vi "VISA_Read_4CHparalelos.vi"() -> ()   [LabVIEW 2019]
uses:
  <vilib>/Instr/_visa.llb/VISA Configure Serial Port (Instr).vi
panel:
  out "Plot 3":dbl[](graph)
  out "Plot 2":dbl[](graph)
  out "Plot 1":dbl[](graph)
  out "Plot 0":dbl[](graph)
  out "Status Read":errorcluster
  out "Buffer Array":dbl[](array[numeric])
  out "Read Buffer":string
  out "Status Serial":errorcluster
  in  "Stop Read":bool
  in  "Start Read":bool
  in  "baud rate (9600)":u32=115200
  in  "data bits (8)":u8=8 min=5 max=8 step=1
  in  "VISA resource name":refnum<visa-resource-name>
  # "Log de Erros"
  # "Conversão Para Inteiro"
  # "Resultado da Leitura"
  # "Controle da porta Serial USB"
  # "Controle da Leitura"
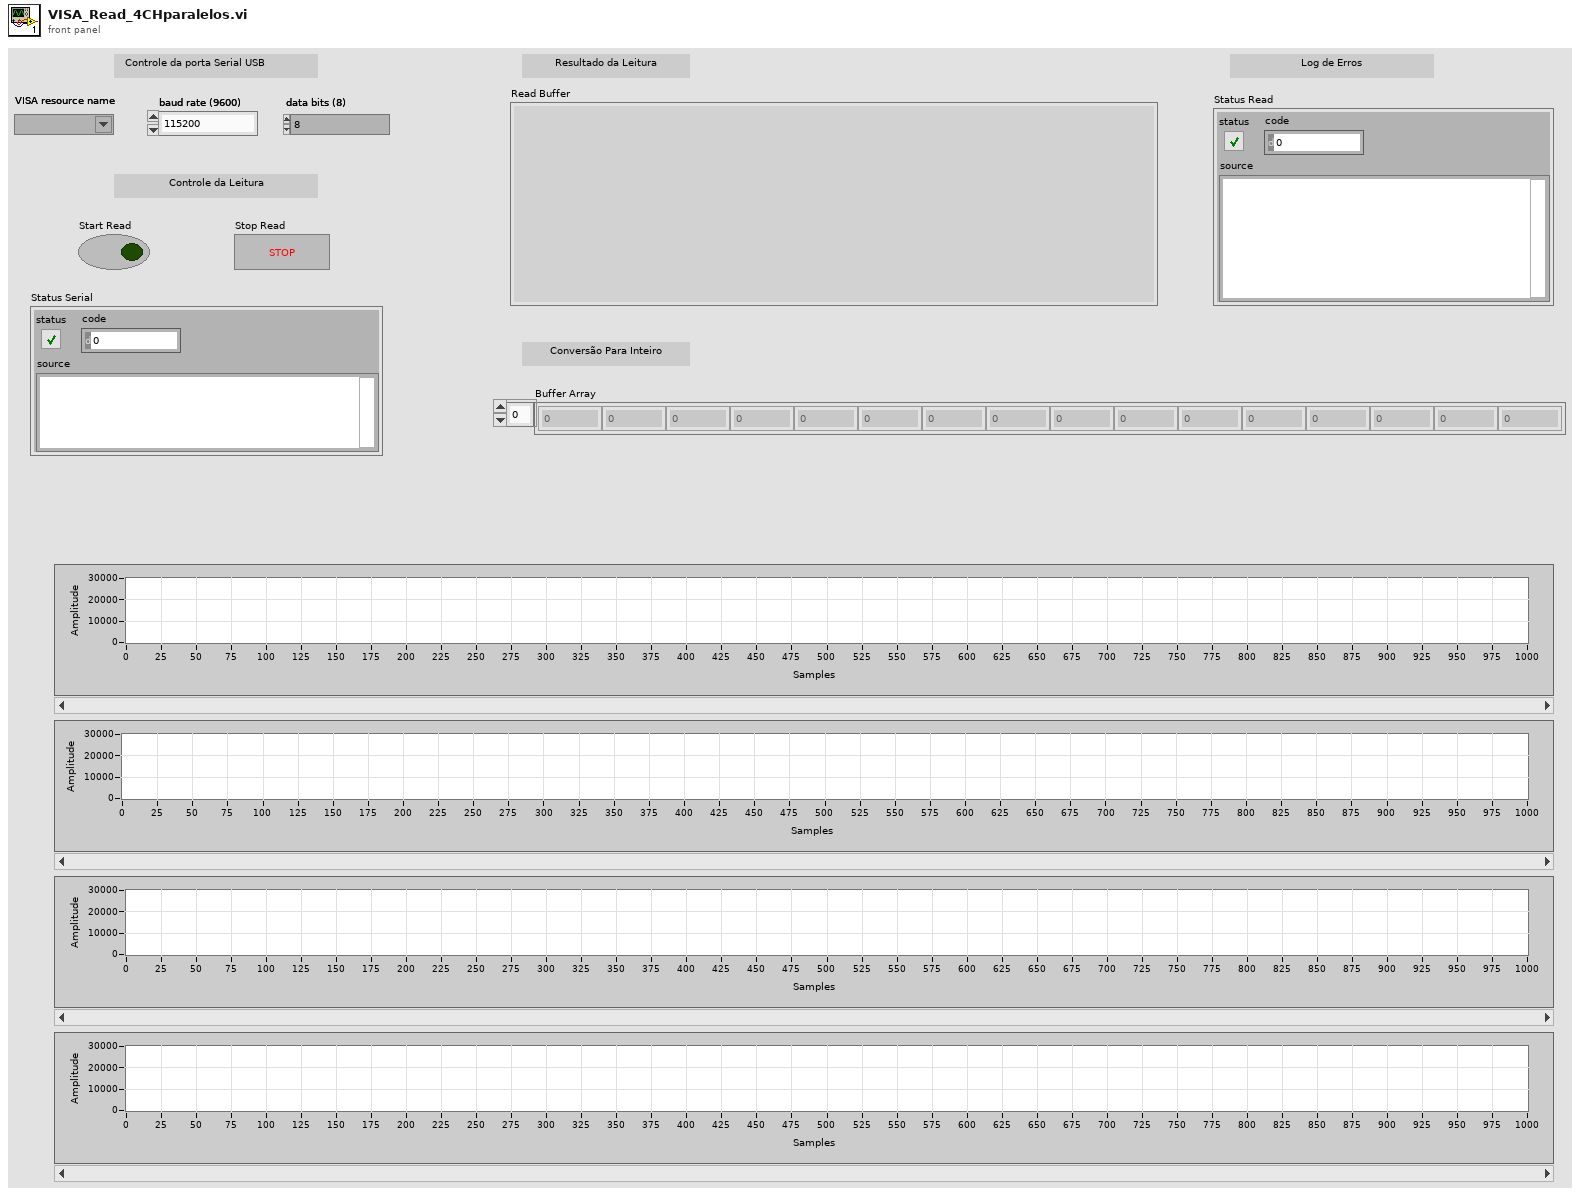
[diagram p1: front panel]
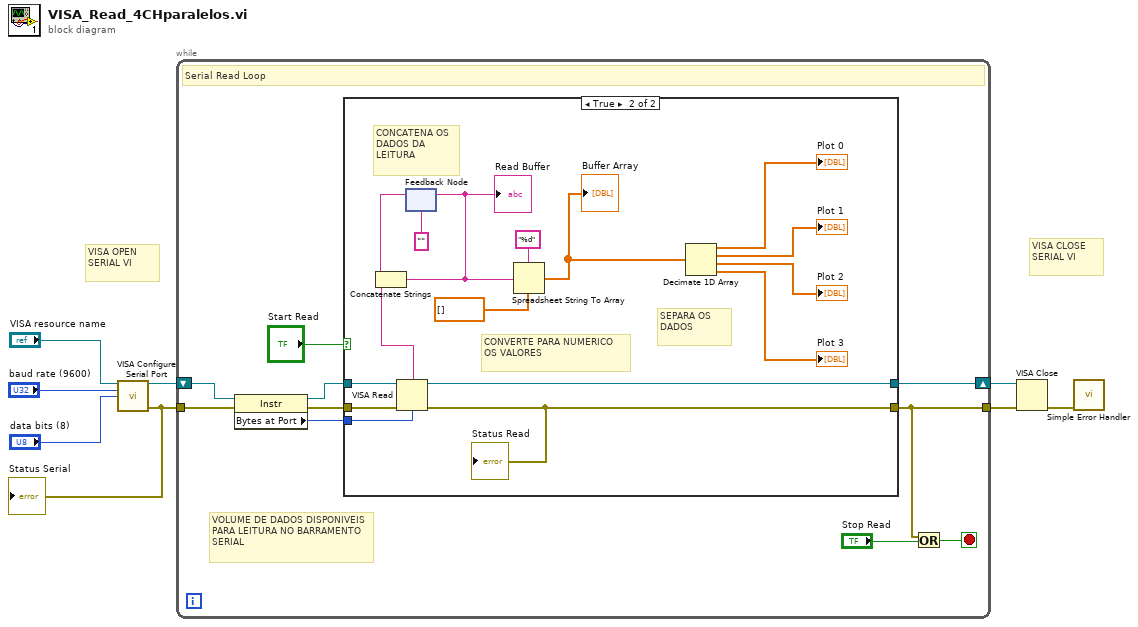
[diagram p0: block diagram]
diagram:
  # "VISA OPEN SERIAL VI"
  # "VISA CLOSE SERIAL VI"
  n1 = call-poly "VISA Configure Serial Port"("VISA resource name"="VISA resource name", "baud rate (9600)"="baud rate (9600)", "data bits (8)"="data bits (8)") -> ("VISA resource name out"=w6:refnum<visa-resource-name>, "error out"=w1:errorcluster)  [unwired: 11 in]
  "Status Serial" <- w1
  n2 = while {
    tunnel: w1 -> [w12]
    tunnel: [w16] -> w7
    shift-right: [w15] -> w5
    shift-left: w6 -> [w13]
    stop <- w14 stop-if-true
    # "VOLUME DE DADOS DISPONIVEIS PARA LEITURA NO BARRAMENTO SERIAL"
    # "Serial Read Loop"
    n3 = property class="Instr"(reference=w13, error in=w12) -> (reference out=w9:refnum<visa-resource-name>, error out=w10:errorcluster, "Bytes at Port"=w11:u32)
    n4 = case shown="True" "Start Read" {
      tunnel: [w19 w36] -> w16
      tunnel: [w20 w33] -> w15
      tunnel: w11 -> [_ w29]
      tunnel: w9 -> [w20 w28]
      tunnel: w10 -> [w19 w27]
      frame False {
        # "OS DADOS SÃO ACUMULADOS NO BUFFER ESPERANDO A PERMISSÃO PARA SER LIDOS"
      }
      frame True {
        # "SEPARA OS DADOS"
        # "CONVERTE PARA NUMERICO OS VALORES"
        # "CONCATENA OS DADOS DA LEITURA"
        n5 = VISA Read(VISA resource name=w28, byte count=w29, error in (no error)=w27) -> (VISA resource name out=w33:refnum<visa-resource-name>, read buffer=w35:string, error out=w36:errorcluster)  [unwired: 1 out]
        "Status Read" <- w36
        n6 = feedback #1("") -> (w30:string)
        n7 = Concatenate Strings(w30, w35) -> (w32:string)
        "Read Buffer" <- w32
        n8 = feedback-in #1(w32) -> ()
        n9 = Spreadsheet String To Array(format string="%d", spreadsheet string=w32, array type (2D Dbl)=dbl[] []) -> (array=w24:dbl[])  [unwired: 1 in]
        "Buffer Array" <- w24
        n10 = Decimate 1D Array(w24) -> (→"Plot 0":dbl[], →"Plot 1":dbl[], →"Plot 2":dbl[], →"Plot 3":dbl[])
      }
    }
    n11 = Or(x=w16, y="Stop Read") -> (x .or. y?=w14:bool)
  }
  n12 = VISA Close(VISA resource name=w5, error in (no error)=w7) -> (error out=w4:errorcluster)
  n13 = call <vilib>:"Simple Error Handler.vi"("error in (no error)"=w4) -> ()  [unwired: 4 in, 5 out]
